vi "iterate.vi"(8 "error in (no error)":errorcluster, 11 "ImagingModeDL090130Frame in":refnum<class "ImagingModeDL090130Frame.lvclass">=refnum) -> (0 "error out":errorcluster, 3 "ImagingModeDL090130Frame out":refnum<class "ImagingModeDL090130Frame.lvclass">)   [LabVIEW 2010, in "ImagingModeDL090130Frame.lvclass"]
uses:
  ImagingModeDL090130Frame.lvclass
  ImagingModeDL090130Frame.lvclass/ImagingModeDL090130Frame.ctl
  common/xcontrols/XIntensityCompensation/XIntensityCompensation/XIntensityCompensation.xctl
  common/classes/ErrorController/ErrorController/class_data.vi
  common/classes/ErrorController/ErrorController/ErrorController.lvclass
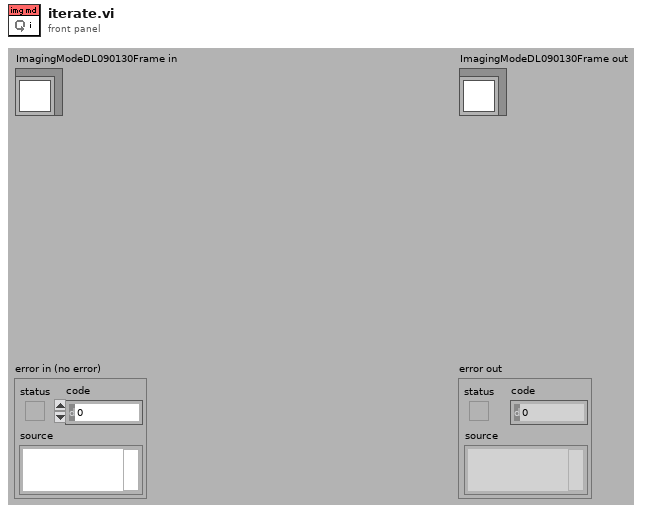
[diagram p1: front panel]
types:
  T1 = typedef "ImagingModeDL090130Frame.lvclass/control_refs.ctl" = cluster{"resolution controls":cluster{"x pixels":refnum<vi>, "y pixels":refnum<vi>, "ratio x factor":refnum<vi>, "ratio y factor":refnum<vi>}, "speed controls":cluster{"pixel dwell time":refnum<vi>, "line scan time":refnum<vi>, "frame rate":refnum<vi>, "keep constant":refnum<vi>}, "number of frames controls":cluster{"# of frames":refnum<vi>, "duration":refnum<vi>, "# of repetitions":refnum<vi>}, "current value indicators":cluster{"frame #":refnum<vi>, "repetition #":refnum<vi>, "offset":refnum<vi>}, "step controls":cluster{"step size":refnum<vi>, "return to origin?":refnum<vi>, "translation mode":refnum<vi>, "XIntensityCompensation":refnum<vi>}, "defineButton":refnum<vi>, "settings enforced?":refnum<vi>, "settings":refnum<vi>}
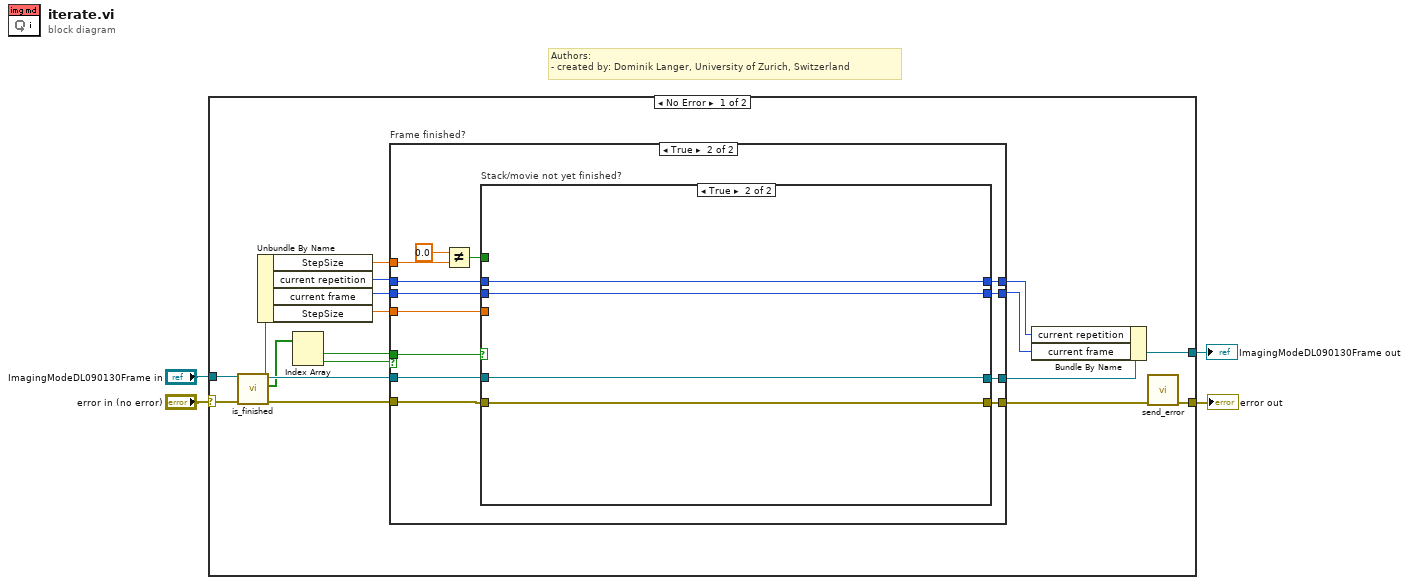
[diagram p0: block diagram]
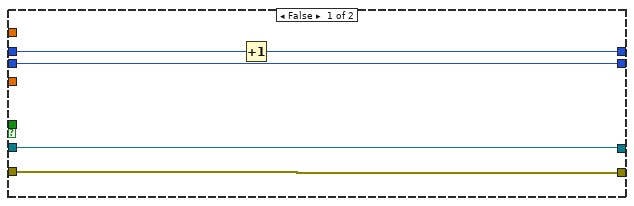
[diagram p2: hidden frame]
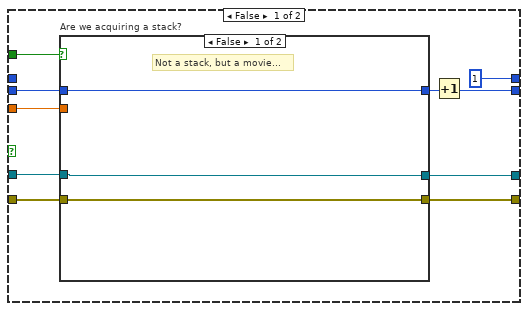
[diagram p3: hidden frame]
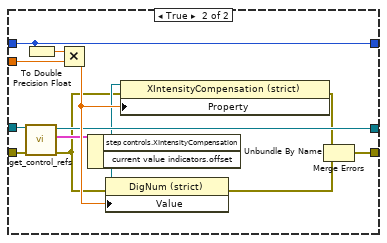
[diagram p4: hidden frame]
diagram:
  # "Authors: \n- created by: Dominik Langer, University of Zurich, Switzerland"
  n1 = case shown="No Error" "error in (no error)" {
    selector: "error in (no error)" -> [w19 w72]
    tunnel: [w20 w72] -> w3
    tunnel: [w18 w71] -> w1
    tunnel: "ImagingModeDL090130Frame in" -> [w21 w71]
    frame No Error {
      n2 = call-dynamic "is_finished.vi"("error in (no error)"=w19, "ImagingModeDL090130Frame in"=w21) -> ("error out"=w7:errorcluster, "finished?"=w9:bool[], "ImagingModeDL090130Frame out"=w11:refnum<class "ImagingModeDL090130Frame.lvclass">)  [unwired: 7 out]
      n3 = Unbundle By Name(w11) -> ("StepSize"=w6:dbl[unit], "current repetition"=w17:i32, "current frame"=w16:i32, "StepSize"=w13:dbl[unit])
      n4 = Index Array(array=w9) -> (element #1=w8:bool, element #2=w10:bool)  [unwired: 2 in]
      n5 = case "Frame finished?" shown="True" w10 {
        tunnel: w17 -> [w26 w27]
        tunnel: [w25 w37] -> w15
        tunnel: w16 -> [w24 w38]
        tunnel: [w24 w39] -> w14
        tunnel: w8 -> [_ w30]
        tunnel: w13 -> [_ w36]
        tunnel: w7 -> [w23 w35]
        tunnel: [w23 w34] -> w5
        tunnel: w11 -> [w22 w33]
        tunnel: [w22 w32] -> w12
        tunnel: w6 -> [_ w31]
        frame False {
          n6 = Increment(x=w26) -> (x+1=w25:i32)
        }
        frame True {
          n7 = Not Equal?(x=dbl[unit] 0.0, y=w31) -> (x != y?=w28:bool)
          n8 = case "Stack/movie not yet finished?" shown="True" w30 {
            tunnel: [w40 w70] -> w39
            tunnel: w38 -> [w48 w70]
            tunnel: [1 w69] -> w37
            tunnel: w27 -> [_ w69]
            tunnel: w36 -> [w47 _]
            tunnel: w35 -> [w44 w68]
            tunnel: [w43 w68] -> w34
            tunnel: w33 -> [w46 w67]
            tunnel: [w45 w67] -> w32
            tunnel: w28 -> [w42 _]
            frame False {
              n9 = case "Are we acquiring a stack?" shown="False" w42 {
                tunnel: w48 -> [w50 w53]
                tunnel: w47 -> [_ w65]
                tunnel: w46 -> [w52 w64]
                tunnel: [w52 w62] -> w45
                tunnel: w44 -> [w51 w56]
                tunnel: [w51 w54] -> w43
                tunnel: [w50 w53] -> w41
                frame False {
                  # "Not a stack, but a movie..."
                }
                frame True {
                  n10 = call-dynamic "get_control_refs.vi"("error in (no error)"=w56, "ImagingModeDL090130Frame in"=w64) -> ("error out"=w55:errorcluster, "control refs"=w61:T1, "ImagingModeDL090130Frame out"=w62:refnum<class "ImagingModeDL090130Frame.lvclass">)  [unwired: 7 in]
                  n11 = To Double Precision Float(number=w53) -> (double precision float=w66:dbl)
                  n12 = Multiply(x=w66, y=w65) -> (x*y=w63:dbl[unit])
                  n13 = Unbundle By Name(w61) -> ("step controls.XIntensityCompensation"=w59:refnum<vi>, "current value indicators.offset"=w60:refnum<vi>)
                  n14 = property class="DigNum (strict)"(reference=w60, error in=w55, "Value"=w63) -> (error out=w58:errorcluster)  [unwired: 1 out]
                  n15 = property class="XIntensityCompensation (strict)"(reference=w59, error in=w55, "Property"=w63) -> (error out=w57:errorcluster)  [unwired: 1 out]
                  n16 = Merge Errors(w57, w58) -> (w54:errorcluster)
                }
              }
              n17 = Increment(x=w41) -> (x+1=w40:i32)
            }
            frame True {
            }
          }
        }
      }
      n18 = Bundle By Name(cluster=w12, "current repetition"=w15, "current frame"=w14) -> (w18:refnum<class "ImagingModeDL090130Frame.lvclass">)
      n19 = call "send_error.vi"("error in (no error)"=w5) -> ("error out"=w20:errorcluster)  [unwired: 10 in]
    }
    frame Error {
    }
  }
  "error out" <- w3
  "ImagingModeDL090130Frame out" <- w1
